vi "BOLA.vi"() -> ()   [LabVIEW 2020]
panel:
  out "Numeric":dbl
  out "Boolean 4":bool
  in  "stop":bool
  out "Boolean 3":bool
  out "Boolean 2":bool
  out "Boolean":bool
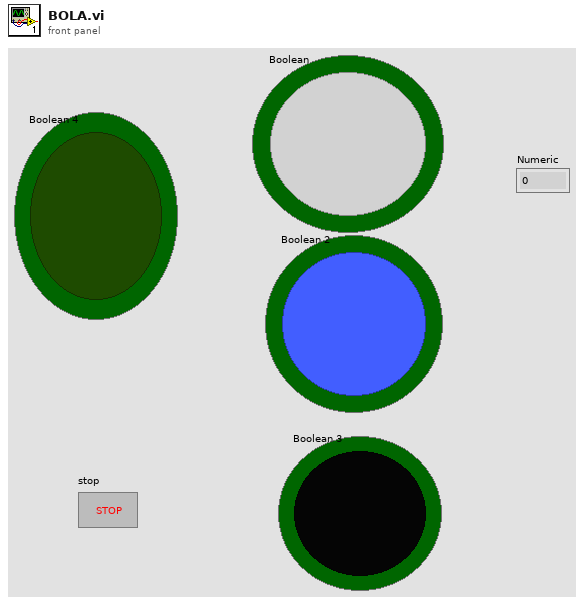
[diagram p1: front panel]
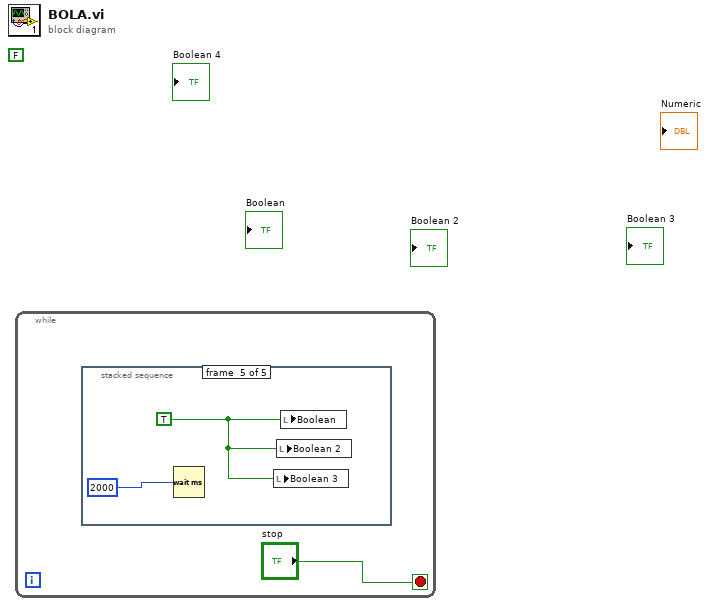
[diagram p0: block diagram]
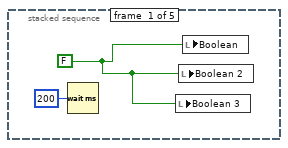
[diagram p2: hidden frame]
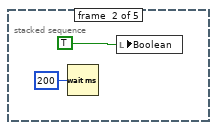
[diagram p3: hidden frame]
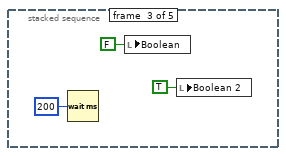
[diagram p4: hidden frame]
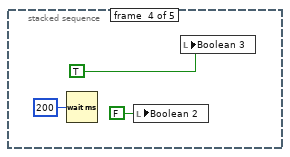
[diagram p5: hidden frame]
diagram:
  (unwired) FALSE
  n1 = while {
    stop <- "stop" stop-if-true
    n2 = stacked-sequence {
      frame #0 {
        w3 = FALSE
        n3 = Wait (ms)(milliseconds to wait=u32 200) -> ()  [unwired: 1 out]
        n4 = local write "Boolean 3"(w3) -> ()
        n5 = local write "Boolean 2"(w3) -> ()
        n6 = local write "Boolean"(w3) -> ()
      }
      frame #1 {
        n7 = Wait (ms)(milliseconds to wait=u32 200) -> ()  [unwired: 1 out]
        n8 = local write "Boolean"(TRUE ("Boolean")) -> ()
      }
      frame #2 {
        n9 = Wait (ms)(milliseconds to wait=u32 200) -> ()  [unwired: 1 out]
        n10 = local write "Boolean"(FALSE ("Boolean")) -> ()
        n11 = local write "Boolean 2"(TRUE ("Boolean 2")) -> ()
      }
      frame #3 {
        n12 = Wait (ms)(milliseconds to wait=u32 200) -> ()  [unwired: 1 out]
        n13 = local write "Boolean 2"(FALSE ("Boolean 2")) -> ()
        n14 = local write "Boolean 3"(TRUE) -> ()
      }
      frame #4 {
        w13 = TRUE ("Boolean")
        n15 = Wait (ms)(milliseconds to wait=u32 2000) -> ()  [unwired: 1 out]
        n16 = local write "Boolean 3"(w13) -> ()
        n17 = local write "Boolean 2"(w13) -> ()
        n18 = local write "Boolean"(w13) -> ()
      }
    }
  }
